vi "CSData_contents.vi"   [LabVIEW 2012]
doc: "Contains all VIs of each Data class that are loaded dynamically during run-time."
uses:
  DiscArchiver/DiscArchiver.lvlib
  EventBuilder/EventBuilder.lvlib
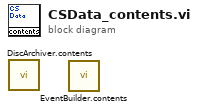
[diagram p0: block diagram]
diagram:
  n1 = call "DiscArchiver.contents.vi"() -> ()  [unwired: 1 in]
  n2 = call "EventBuilder.contents.vi"() -> ()  [unwired: 1 in]
